vi "Latihan 1 (Cerdas Cermat).vi"() -> ()   [LabVIEW 2021]
panel:
  out "Buzzer":bool
  out "Lampu 4":bool
  out "Lampu 3":bool
  out "Lampu 2":bool
  out "Lampu 1":bool
  in  "D":bool
  in  "C":bool
  in  "B":bool
  in  "A":bool
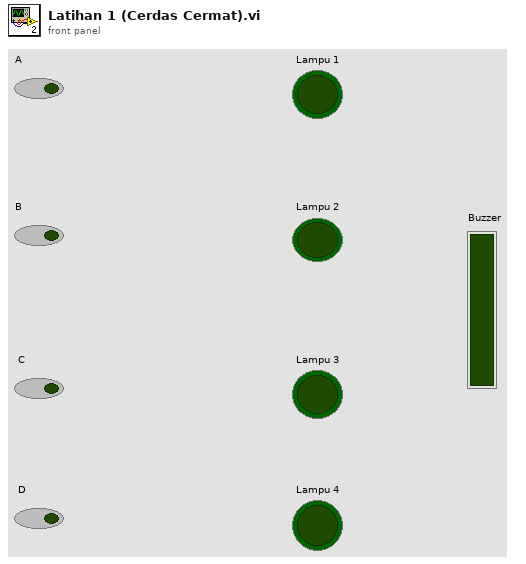
[diagram p1: front panel]
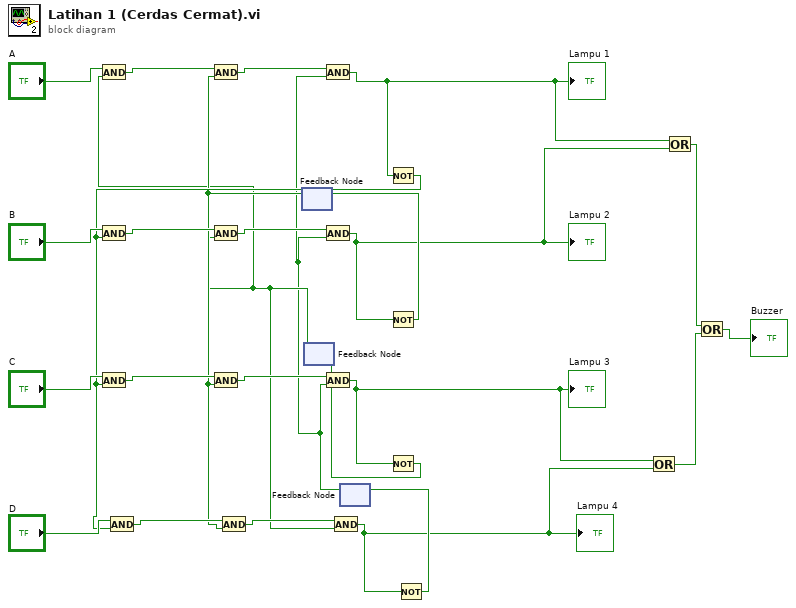
[diagram p0: block diagram]
diagram:
  n1 = feedback #1() -> (w12:bool)  [unwired: 1 in]
  n2 = feedback #2() -> (w10:bool)  [unwired: 1 in]
  n3 = And(x="A", y=w10) -> (x .and. y?=w25:bool)
  n4 = And(x=w25, y=w12) -> (x .and. y?=w24:bool)
  n5 = feedback #3() -> (w8:bool)  [unwired: 1 in]
  n6 = And(x=w24, y=w8) -> (x .and. y?=w7:bool)
  "Lampu 1" <- w7
  n7 = Not(x=w7) -> (.not. x?=w14:bool)
  n8 = And(x="B", y=w14) -> (x .and. y?=w22:bool)
  n9 = And(x="C", y=w14) -> (x .and. y?=w19:bool)
  n10 = And(x="D", y=w14) -> (x .and. y?=w16:bool)
  n11 = And(x=w22, y=w10) -> (x .and. y?=w21:bool)
  n12 = And(x=w19, y=w12) -> (x .and. y?=w18:bool)
  n13 = And(x=w16, y=w12) -> (x .and. y?=w15:bool)
  n14 = And(x=w21, y=w8) -> (x .and. y?=w6:bool)
  "Lampu 2" <- w6
  n15 = And(x=w18, y=w8) -> (x .and. y?=w5:bool)
  "Lampu 3" <- w5
  n16 = And(x=w15, y=w10) -> (x .and. y?=w4:bool)
  "Lampu 4" <- w4
  n17 = Not(x=w6) -> (.not. x?=w13:bool)
  n18 = feedback-in #1(w13) -> ()
  n19 = Not(x=w5) -> (.not. x?=w11:bool)
  n20 = feedback-in #2(w11) -> ()
  n21 = Not(x=w4) -> (.not. x?=w9:bool)
  n22 = feedback-in #3(w9) -> ()
  n23 = Or(x=w5, y=w4) -> (x .or. y?=w3:bool)
  n24 = Or(x=w7, y=w6) -> (x .or. y?=w2:bool)
  n25 = Or(x=w2, y=w3) -> (x .or. y?=→"Buzzer":bool)
